vi "Initialize.vi"(8 "error in":errorcluster, 10 "parameters":variant, 11 "node in":refnum<class "E2E Tag Exchange editor node.lvclass">) -> (0 "error out":errorcluster, 2 "summary":T2[](array[typedef]), 3 "data value reference":T1)   [LabVIEW 2015, in "E2E Tag Exchange editor node.lvclass"]
doc: "Initializes the data of a node to its default state.\nThe object is not created inside of this VI, because it is created from a File depending on user selection.\nCopyright 2015 National Instruments Corporation\n\nLicensed under the Apache License, Version 2.0 (the \"License\"); you may not use this file except in compliance with the License. You may obtain a copy of the License at http://www.apache.org/licenses/LICENSE-2.0\nUnless required by applicable law or agreed to in writing, software distributed under the License is distributed on an \"AS IS\" BASIS, WITHOUT WARRANTIES OR CONDITIONS OF ANY KIND, either express or implied. See the License for the specific language governing permissions and limitations under the License."
uses:
  E2E Tag Exchange editor node.lvclass
  <vilib>/NI/Configuration Framework/Node/Summary.ctl
  <vilib>/NI/Configuration Framework/Node/NodeRef.ctl
  <vilib>/NI/Configuration Framework/Node/NISE_CEF_Node.lvclass
  Node LUT/Command.ctl
  <vilib>/NI/DCAF/Tag Editor Core/Configuration Editor/Classes/Module editor node/module editor node.lvclass
  Node LUT/Node LUT.lvlib
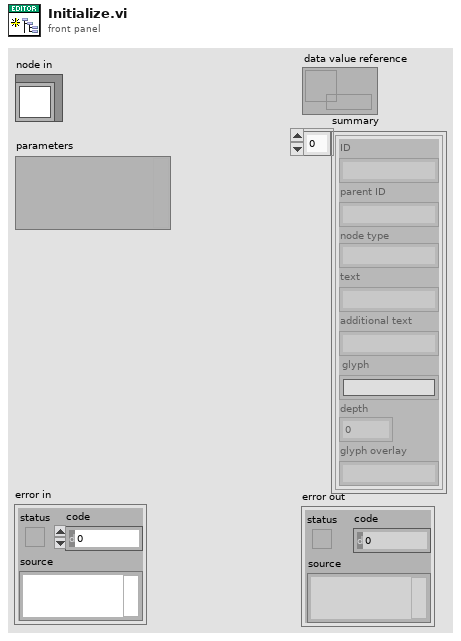
[diagram p1: front panel]
types:
  T1 = typedef "NISE_CEF_Node.lvclass/NodeRef.ctl" = refnum<data-value>
  T2 = typedef "NISE_CEF_Node.lvclass/Summary.ctl" = cluster{"ID":string, "parent ID":string, "node type":string, "text":string, "additional text":string, "glyph":string, "depth":i32, "glyph overlay":string}
  T3 = typedef "Node LUT.lvlib/Command.ctl" = enum16{"Initialize", "Add Node", "Remove Node", "Node Ref from UID", "List Nodes"}
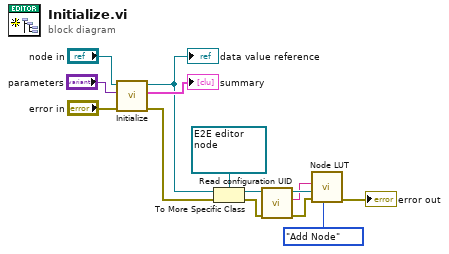
[diagram p0: block diagram]
diagram:
  n1 = call-parent "Initialize.vi"("error in"="error in", "parameters"="parameters", "node in"="node in") -> ("error out"=w2:errorcluster, "summary"=→"summary":T2[], "data value reference"=w3:T1)  [unwired: 6 in]
  "data value reference" <- w3
  n2 = To More Specific Class(target class=refnum<data-value> refnum, reference=w3, error in=w2) -> (specific class reference=w9:refnum<data-value>, error out=w5:errorcluster)
  n3 = call "Read configuration UID.vi"("error in (no error)"=w5, "E2E editor node in"=w9) -> ("error out"=w7:errorcluster, "Module UID"=w6:string, "E2E editor node out"=w10:refnum<data-value>)  [unwired: 7 in]
  n4 = call "Node LUT.vi"("Command"=Command."Add Node", "error in"=w7, "node ref"=w10, "UID"=w6) -> ("error out"=→"error out":errorcluster)  [unwired: 4 in, 3 out]
